vi "9213_Initialize.vi"(7 "Module Model":T1=enum."NI 9205", 8 "error in (no error)":errorcluster, 9 "Slot Settings":T2, 11 "9213 in":refnum<class "9213.lvclass">) -> (0 "error out":errorcluster, 3 "9213 out":refnum<class "9213.lvclass">)   [LabVIEW 2017, in "Modules.lvlib" / "9213.lvclass"]
uses:
  9213.lvclass
  RSI Module/Slot Settings.ctl
  C:/Users/dbuck/Documents/GitHub/Scan-Engine-Custom-Device-Classes/Source/RSI Module/RSI Module.lvclass
  RSI Module/Module Models.ctl
  RSI Module/Channels.ctl
  RSI Module/Channel Type.ctl
  Conversion Time.ctl
  Measurement Units.ctl
  Thermocouple Type.ctl
  9213.lvclass/9213.ctl
  RSI Module/RSI Module.lvclass
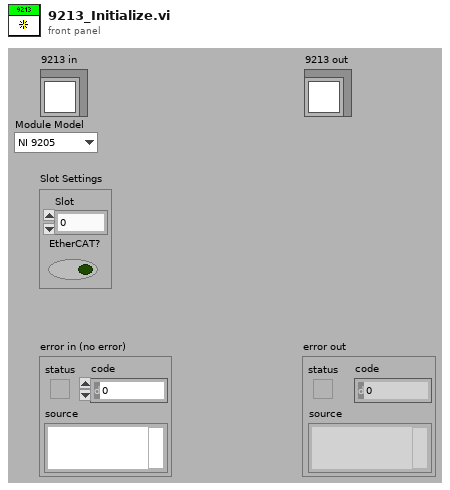
[diagram p1: front panel]
types:
  T1 = typedef "Modules.lvlib/RSI Module.lvclass/Module Models.ctl" = enum16{"Empty", "NI 9201", "NI 9203", "NI 9205", "NI 9206", "NI 9207", "NI 9208", "NI 9211", "NI 9212", "NI 9213", "NI 9214", "NI 9215", "NI 9217", "NI 9219", "NI 9220", "NI 9221", "NI 9222", "NI 9223", "NI 9225", "NI 9227", "NI 9229", "NI 9233", "NI 9234", "NI 9235", "NI 9236", "NI 9237", "NI 9239", "NI 9242", "NI 9244", "NI 9263", "NI 9264", "NI 9265", "NI 9269", "NI 9375", "NI 9401", "NI 9402", "NI 9403", "NI 9411", "NI 9421", "NI 9422", "NI 9423", "NI 9425", "NI 9426", "NI 9435", "NI 9437", "NI 9472", "NI 9474", "NI 9475", "NI 9476", "NI 9477", "NI 9478", "NI 9481", "NI 9482", "NI 9485"}
  T2 = typedef "Modules.lvlib/RSI Module.lvclass/Slot Settings.ctl" = cluster{"Slot":u32, "EtherCAT?":bool}
  T3 = typedef "Modules.lvlib/9213.lvclass/Conversion Time.ctl" = u16
  T4 = typedef "Modules.lvlib/RSI Module.lvclass/Channels.ctl" = cluster{"# Input Channels":i32, "# Output Channels":i32, "Channel Type":T5, "Units":string}
  T5 = typedef "Modules.lvlib/RSI Module.lvclass/Channel Type.ctl" = enum16{"Analog", "Digital"}
  T6 = typedef "Modules.lvlib/9213.lvclass/Thermocouple Type.ctl" = u8
  T7 = typedef "Modules.lvlib/9213.lvclass/Measurement Units.ctl" = u8
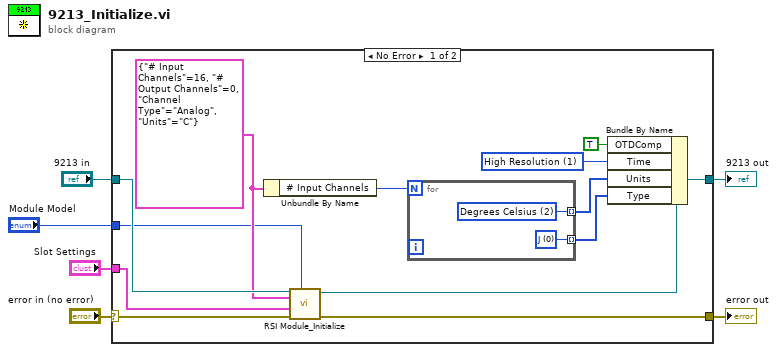
[diagram p0: block diagram]
diagram:
  n1 = case shown="No Error" "error in (no error)" {
    selector: "error in (no error)" -> [w17 w23]
    tunnel: [w16 w23] -> w5
    tunnel: [w14 w22] -> w3
    tunnel: "9213 in" -> [w19 w22]
    tunnel: "Slot Settings" -> [w18 _]
    tunnel: "Module Model" -> [w8 _]
    frame No Error {
      w13 = T3 1 items=["High Speed", "High Resolution"] ("Time")
      w12 = T4 {"# Input Channels"=16, "# Output Channels"=0, "Channel Type"=enum."Analog", "Units"="C"} ("Channels")
      n2 = Unbundle By Name(w12) -> ("# Input Channels"=w11:i32)
      n3 = call "RSI Module_Initialize.vi"("Module Model"=w8, "error in (no error)"=w17, "Slot Settings"=w18, "Channels"=w12, "RSI Module in"=w19) -> ("error out"=w16:errorcluster, "RSI Module out"=w15:refnum<class "9213.lvclass">)  [unwired: 5 in]
      n4 = for {
        N: w11 -> [_]
        tunnel: [w21] -> w10 mode=indexing
        tunnel: [w20] -> w9 mode=indexing
        w20 = T6 0 items=["J", "K", "T", "E", "R", "S", "N", "B"] ("Type")
        w21 = T7 2 items=["Raw Volts", "Degrees Kelvin", "Degrees Celsius", "Degrees Fahrenheit", "Degrees Rankine"] ("Units")
      }
      n5 = Bundle By Name(cluster=w15, "OTDComp"=TRUE, "Time"=w13, "Units"=w10, "Type"=w9) -> (w14:refnum<class "9213.lvclass">)
    }
    frame Error {
    }
  }
  "error out" <- w5
  "9213 out" <- w3
